vi "短信服务全局变量.vi"() -> ()   [LabVIEW 2016]
panel:
  in  "启用":bool
  in  "站点":string
  in  "PhoneNumbers":string
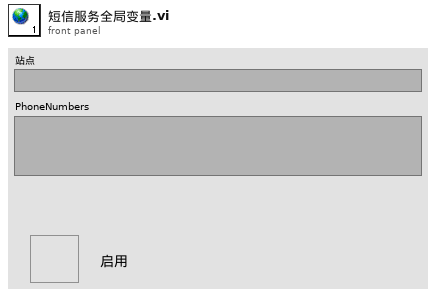
[diagram p1: front panel]
diagram:
